vi "ParseFpgaconfigXml.vi"(8 "error in (no error)":errorcluster, 11 "Path":path=path "C:/_git/FlexLogger-RioStreamer/fpga/R Series Example.fpgaconfig") -> (0 "error out":errorcluster, 3 "data":T1)   [LabVIEW 2024, in "RIO Streamer.lvlib" / "FIFO Reader.lvclass"]
uses:
  FIFO Reader.lvclass
  NiVeriStandFpgaDmaXml.ctl
  PacketInfo.ctl
  <vilib>/xml/Close Reference(Node).vi
  FIFO Reader.lvclass/FIFO Reader.ctl
  <vilib>/xml/Load XML File.vi
  <vilib>/xml/NI_XML.lvlib
  <resource>/objmgr/DOMUserDefRef.rc
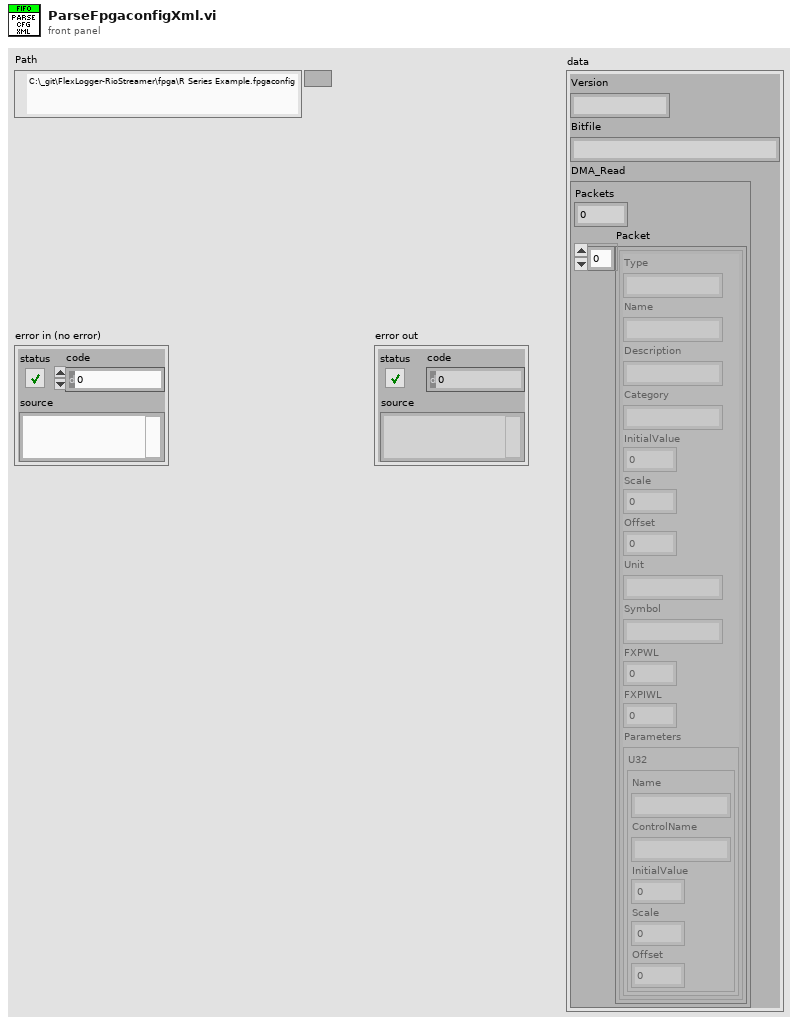
[diagram p1: front panel]
types:
  T1 = typedef "RIO Streamer.lvlib/FIFO Reader.lvclass/NiVeriStandFpgaDmaXml.ctl" = cluster{"Version":string, "Bitfile":string, "DMA_Read":cluster{"Packets":i32, "Packet":T2[]}}
  T2 = typedef "RIO Streamer.lvlib/FIFO Reader.lvclass/PacketInfo.ctl" = cluster{"Type":string, "Name":string, "Description":string, "Category":string, "InitialValue":dbl, "Scale":dbl, "Offset":dbl, "Unit":string, "Symbol":string, "FXPWL":i16, "FXPIWL":i16, "Parameters":cluster{"U32":cluster{"Name":string, "ControlName":string, "InitialValue":dbl, "Scale":dbl, "Offset":dbl}}}
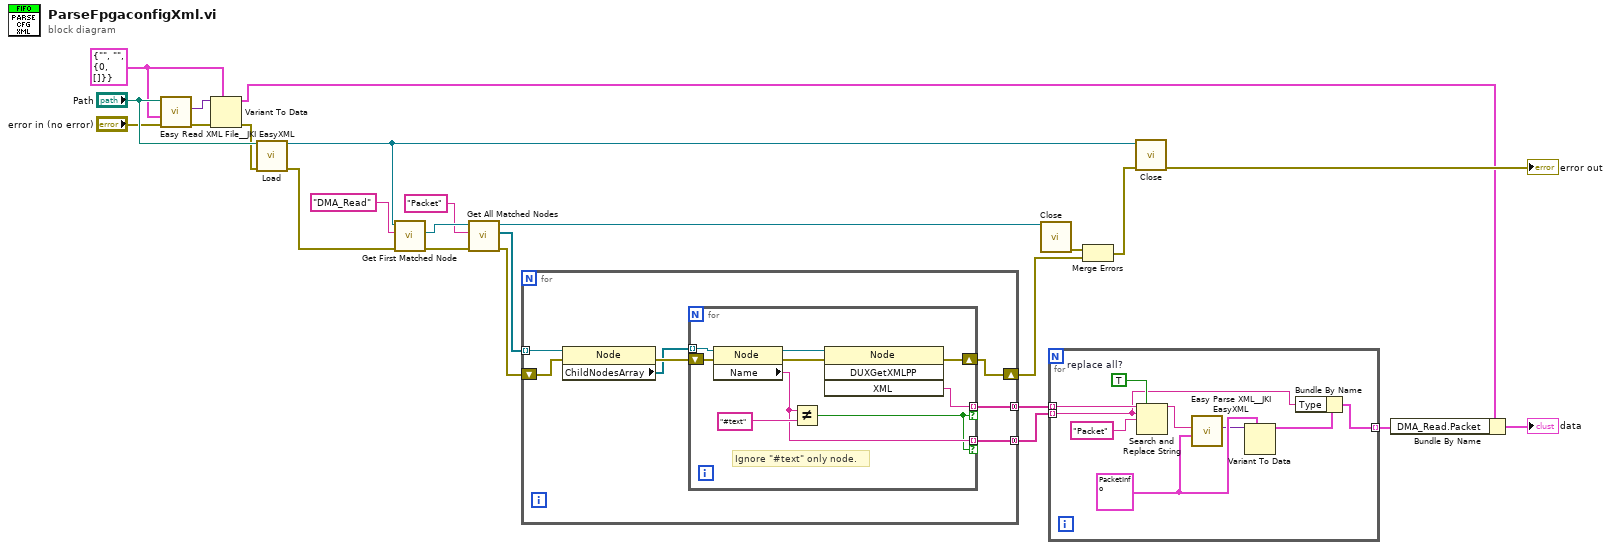
[diagram p0: block diagram]
diagram:
  w13 = T1 {"Version"="", "Bitfile"="", "DMA_Read"={"Packets"=0, "Packet"=[]}} ("FPGADMAChannelData")
  n1 = call <vilib>:"Easy Read XML File__JKI EasyXML.vi"("error in (no error)"="error in (no error)", "LabVIEW Data (Type)"=w13, "XML File Path"="Path") -> ("error out"=w12:errorcluster, "LabVIEW Data"=w14:variant)  [unwired: 6 in, 1 out]
  n2 = Variant To Data(error in=w12, type=w13, Variant=w14) -> (data=w9:T1, error out=w10:errorcluster)
  n3 = call-poly <vilib>:"Load.vi"("path to XML document"="Path", "error in (no error)"=w10) -> ("DOM document out"=w16:refnum<k20>, "error out"=w8:errorcluster)  [unwired: 11 in, 1 out]
  n4 = call <vilib>:"Get First Matched Node.vi"("error in (no error)"=w8, "XPath expression"="DMA_Read", "node in"=w16) -> ("error out"=w21:errorcluster, "node result"=w20:refnum<k20>)  [unwired: 6 in, 1 out]
  n5 = call <vilib>:"Get All Matched Nodes.vi"("error in (no error)"=w21, "XPath expression"="Packet", "node in"=w20) -> ("error out"=w6:errorcluster, "node result array"=w7:refnum<k20>[], "node out"=w18:refnum<k20>)  [unwired: 6 in]
  n6 = for {
    tunnel: w7 -> [w26] mode=indexing
    shift-right: [w31] -> w5
    shift-left: w6 -> [w30]
    tunnel: [w27] -> w4 mode=concatenating
    tunnel: [w25] -> w3 mode=concatenating
    n7 = property class="Node"(reference=w26, error in=w30) -> (error out=w29:errorcluster, "ChildNodesArray"=w28:refnum<k20>[])  [unwired: 1 out]
    n8 = for {
      shift-right: [w38] -> w31
      shift-left: w29 -> [w37]
      tunnel: w28 -> [w36] mode=indexing
      tunnel: [w35] -> w27 mode=indexing if=w32
      tunnel: [w33] -> w25 mode=indexing if=w32
      # "Ignore \"#text\" only node."
      n9 = property class="Node"(reference=w36, error in=w37) -> (reference out=w40:refnum<k20>, error out=w39:errorcluster, "Name"=w33:string)
      n10 = Not Equal?(x=w33, y="#text") -> (x != y?=w32:bool)
      n11 = invoke class="Node" method="DUXGetXMLPP"(reference=w40, error in=w39) -> (error out=w38:errorcluster, "XML"=w35:string)  [unwired: 2 in, 2 out]
    }
  }
  n12 = call-poly <vilib>:"Close.vi"("node"=w18) -> ("error out"=w17:errorcluster)  [unwired: 8 in]
  n13 = for {
    tunnel: w4 -> [w49] mode=indexing
    tunnel: w3 -> [w42] mode=indexing
    tunnel: [w41] -> w2 mode=indexing
    w44 = TRUE  # replace all?
    w47 = T2 {"Type"="", "Name"="", "Description"="", "Category"="", "InitialValue"=0.0, "Scale"=0.0, "Offset"=0.0, "Unit"="", "Symbol"="", "FXPWL"=0, "FXPIWL"=0, "Parameters"={"U32"={"Name"="", "ControlName"="", "InitialValue"=0.0, "Scale"=0.0, "Offset"=0.0}}} ("Packet Info")
    n14 = Search and Replace String(replace all?=w44, input string=w49, search string=w42, replace string="Packet" ("replace string (\"\")")) -> (result string=w45:string)  [unwired: 4 in, 3 out]
    n15 = call <vilib>:"Easy Parse XML__JKI EasyXML.vi"("LabVIEW Data (Type)"=w47, "XML String"=w45) -> ("LabVIEW Data"=w46:variant)  [unwired: 8 in, 1 out]
    n16 = Variant To Data(type=w47, Variant=w46) -> (data=w43:T2)  [unwired: 1 in, 1 out]
    n17 = Bundle By Name(cluster=w43, "Type"=w42) -> (w41:T2)
  }
  n18 = Merge Errors(w17, w5) -> (w22:errorcluster)
  n19 = call-poly <vilib>:"Close.vi"("error in (no error)"=w22, "node"=w16) -> ("error out"=→"error out":errorcluster)  [unwired: 7 in]
  n20 = Bundle By Name(cluster=w9, "DMA_Read.Packet"=w2) -> (→"data":T1)
